vi "Create Wheel Object.vi"(8 "error out 2":errorcluster, 10 "Array":T2[](array[typedef]) format="%.0x", 11 "Numeric":u8) -> (0 "error out":errorcluster, 3 "Array 2":T1[](array[typedef]))   [LabVIEW 2023, in "Vires VTD System Explorer.lvlib"]
uses:
  Vires VTD System Explorer.lvlib
  <vilib>/NI VeriStand/Custom Device API/Custom Device Item Ref.ctl
  RDB/RDB Player Object.ctl
  <vilib>/NI VeriStand/Custom Device API/Get Item Property (Variant).vi
  <vilib>/NI VeriStand/Custom Device API/Custom Device API.lvlib
  RDB/RDB.lvlib
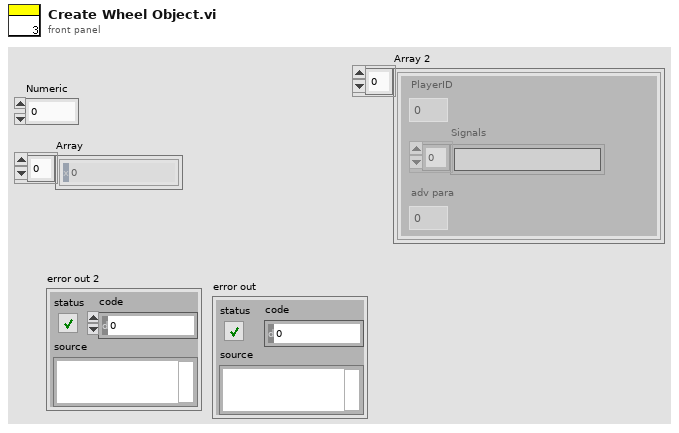
[diagram p1: front panel]
types:
  T1 = typedef "RDB.lvlib/RDB Player Object.ctl" = cluster{"PlayerID":i32, "Signals":string[], "adv para":i32}
  T2 = typedef "Custom Device API.lvlib/Custom Device Item Ref.ctl" = u64
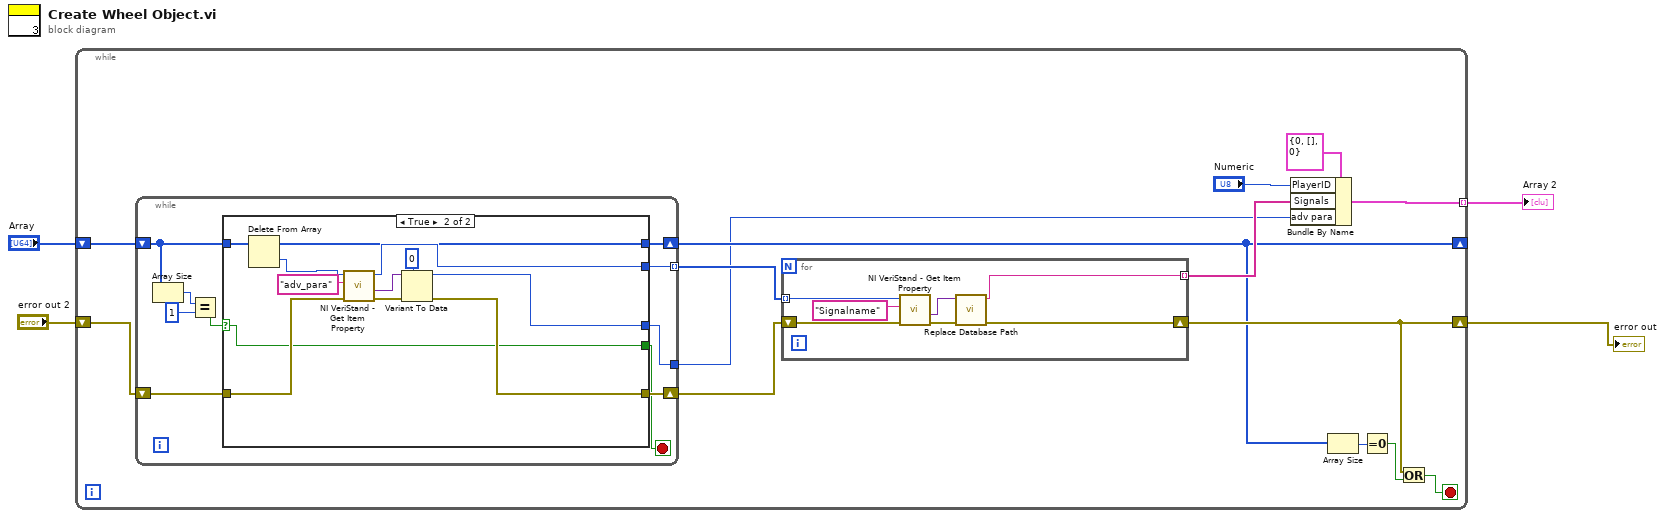
[diagram p0: block diagram]
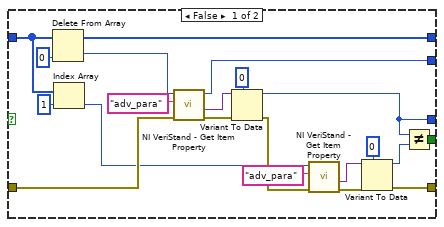
[diagram p2: hidden frame]
diagram:
  n1 = while {
    shift-right: [w7] -> w3
    shift-left: "error out 2" -> [w12]
    tunnel: [w11] -> w2 mode=indexing
    shift-right: [w6] -> _
    shift-left: "Array" -> [w15]
    stop <- w8 stop-if-true
    n2 = while {
      shift-right: [w28] -> w13
      shift-left: w12 -> [w27]
      tunnel: [w25] -> w14 mode=indexing
      tunnel: [w24] -> w5
      shift-right: [w19] -> w6
      shift-left: w15 -> [w21]
      stop <- w26 stop-if-true
      n3 = Array Size(array=w21) -> (size(s)=w22:i32)
      n4 = Equal?(x=w22, y=1) -> (x = y?=w20:bool)
      n5 = case shown="True" w20 {
        selector: w20 -> [_ w55]
        tunnel: [w42 w56] -> w28
        tunnel: w27 -> [w41 w57]
        tunnel: [w37 w55] -> w26
        tunnel: [w36 w54] -> w25
        tunnel: [w35 w53] -> w24
        tunnel: w21 -> [w34 w52]
        tunnel: [w29 w51] -> w19
        frame False {
          n6 = Delete From Array(array=w34, index=0) -> (deleted portion=w30:T2, array with subset deleted=w29:T2[])  [unwired: 1 in]
          n7 = Index Array(array=w34, index=1) -> (element=w33:T2)
          n8 = call-poly <vilib>:"NI VeriStand - Get Item Property.vi"("error in (no error)"=w41, "Property Name"="adv_para", "Item Ref in"=w30) -> ("error out"=w47:errorcluster, "Value"=w46:variant, "Item Ref out"=w36:T2)  [unwired: 5 in, 1 out]
          n9 = Variant To Data(error in=w47, type=u8 0, Variant=w46) -> (data=w35:u8, error out=w45:errorcluster)
          n10 = call-poly <vilib>:"NI VeriStand - Get Item Property.vi"("error in (no error)"=w45, "Property Name"="adv_para", "Item Ref in"=w33) -> ("error out"=w44:errorcluster, "Value"=w43:variant)  [unwired: 5 in, 2 out]
          n11 = Variant To Data(error in=w44, type=u8 0, Variant=w43) -> (data=w39:u8, error out=w42:errorcluster)
          n12 = Not Equal?(x=w35, y=w39) -> (x != y?=w37:bool)
        }
        frame True {
          n13 = Delete From Array(array=w52) -> (deleted portion=w50:T2, array with subset deleted=w51:T2[])  [unwired: 2 in]
          n14 = call-poly <vilib>:"NI VeriStand - Get Item Property.vi"("error in (no error)"=w57, "Property Name"="adv_para", "Item Ref in"=w50) -> ("error out"=w59:errorcluster, "Value"=w60:variant, "Item Ref out"=w54:T2)  [unwired: 5 in, 1 out]
          n15 = Variant To Data(error in=w59, type=u8 0, Variant=w60) -> (data=w53:u8, error out=w56:errorcluster)
        }
      }
    }
    n16 = for {
      tunnel: w14 -> [w64] mode=indexing
      shift-right: [w62] -> w7
      shift-left: w13 -> [w65]
      tunnel: [w63] -> w16 mode=indexing
      n17 = call-poly <vilib>:"NI VeriStand - Get Item Property.vi"("error in (no error)"=w65, "Property Name"="Signalname", "Item Ref in"=w64) -> ("error out"=w67:errorcluster, "Value"=w68:variant)  [unwired: 5 in, 2 out]
      n18 = call "Replace Database Path.vi"("error in (no error)"=w67, "Value"=w68) -> ("error out"=w62:errorcluster, "Property Name"=w63:string)  [unwired: 8 in]
    }
    n19 = Bundle By Name(cluster=T1 {"PlayerID"=0, "Signals"=[], "adv para"=0} ("RDB Player Objects"), "PlayerID"="Numeric", "Signals"=w16, "adv para"=w5) -> (w11:T1)
    n20 = Array Size(array=w6) -> (size(s)=w9:i32)
    n21 = Equal To 0?(x=w9) -> (x = 0?=w10:bool)
    n22 = Or(x=w7, y=w10) -> (x .or. y?=w8:bool)
  }
  "error out" <- w3
  "Array 2" <- w2
